vi "Untitled 9vi.vi"() -> ()   [LabVIEW 2009]
uses:
  <vilib>/Utility/file.llb/Read From Spreadsheet File (DBL).vi
  <vilib>/Analysis/NI_AALBase.lvlib
panel:
  in  "method":i32(ring)=1 items=["median", "noise center", "Minimum", "lower 20th"]
  out "white peaks":dbl
  out "white peaks normed":dbl
  out "red peaks normed":dbl
  in  "butterworth?":bool
  in  "w":dbl
  out "red peaks":dbl
  out "output cluster 3":cluster{"locations":dbl[], "locations":dbl[]}(graph)
  out "output cluster 2":cluster{"locations":dbl[], "amplitudes":dbl[]}[](graph)
  in  "threshold":dbl
  in  "number of rows (all:-1)":i32=300
  out "all rows":dbl[][](graph)
  in  "file path (dialog if empty)":path
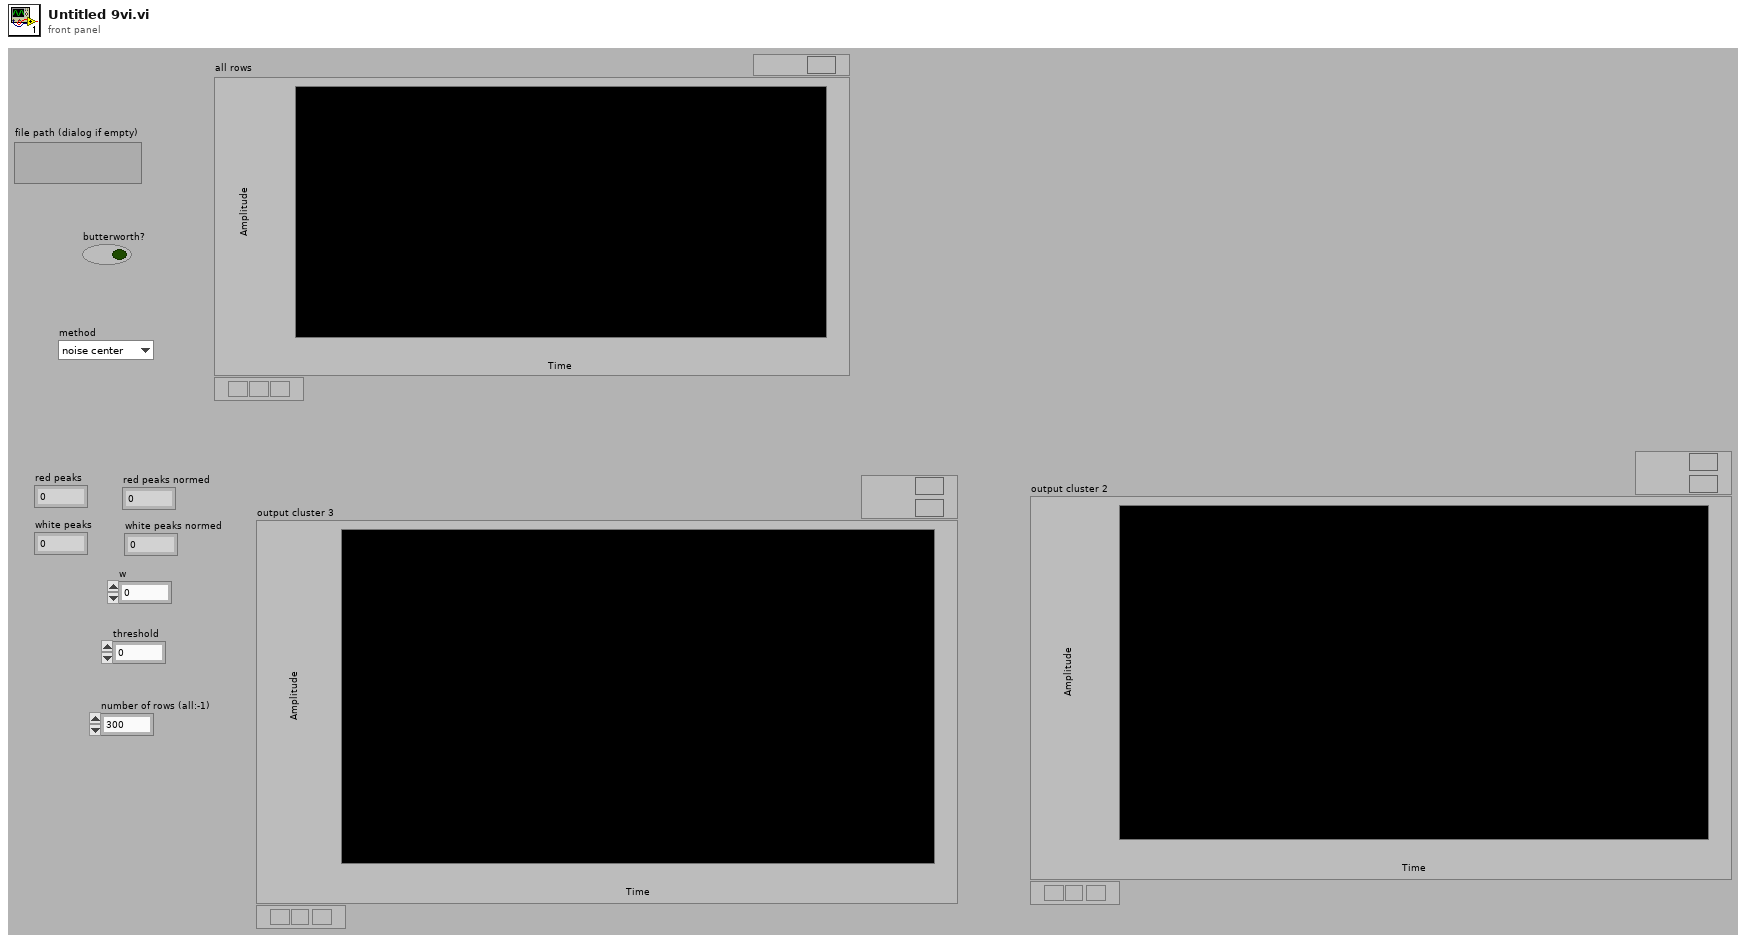
[diagram p1: front panel]
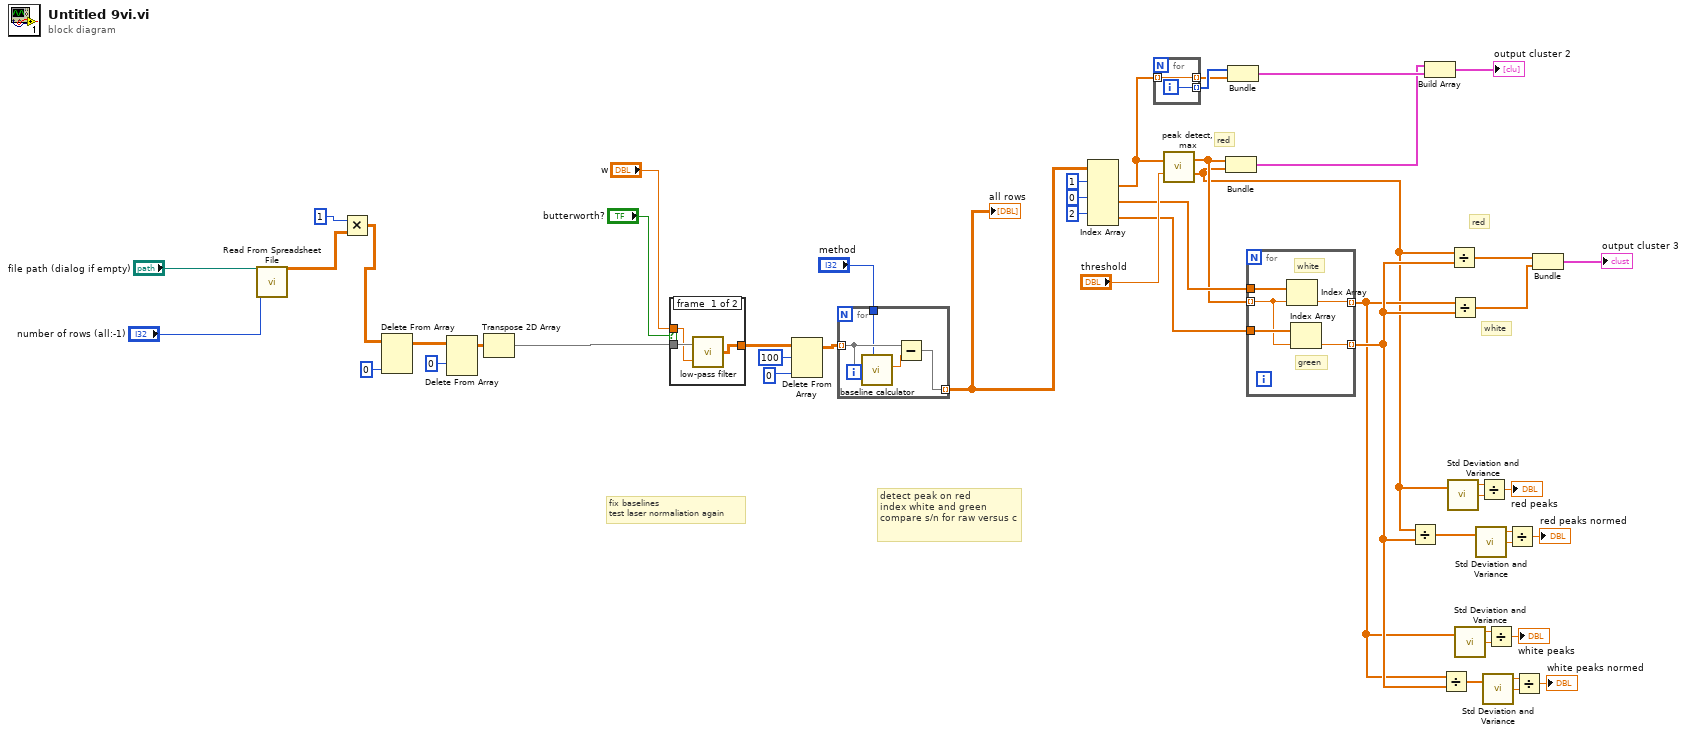
[diagram p0: block diagram]
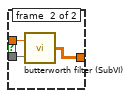
[diagram p2: hidden frame]
diagram:
  # "white"
  # "red"
  # "red"
  # "detect peak on red\nindex white and green\ncompare s/n for raw versus c"
  # "fix baselines\ntest laser normaliation again"
  n1 = call-poly <vilib>:"Read From Spreadsheet File.vi"("number of rows (all:-1)"="number of rows (all:-1)", "file path (dialog if empty)"="file path (dialog if empty)") -> ("all rows"=w44:dbl[][])  [unwired: 5 in, 4 out]
  n2 = Multiply(x=1 ("disabled index (col)"), y=w44) -> (x*y=w43:dbl[][])
  n3 = Delete From Array(array=w43, index (col)=0 ("disabled index (col)")) -> (array with subset deleted=w47:dbl[][])  [unwired: 2 in, 1 out]
  n4 = Delete From Array(array=w47, index (row)=0 ("disabled index (col)")) -> (array with subset deleted=w46:dbl[][])  [unwired: 2 in, 1 out]
  n5 = Transpose 2D Array(2D array=w46) -> (transposed array=w26:dbl[][])
  n6 = case shown="True" "butterworth?" {
    tunnel: "w" -> [w53 w57]
    tunnel: w26 -> [w54 w56]
    tunnel: [w52 w55] -> w12
    frame #0 {
      n7 = call "low-pass filter.vi"("smooth size"=w53, "Array 2"=w54) -> ("Array"=w52:dbl[][])
    }
    frame #1 {
      n8 = call "butterworth filter (SubVI).vi"("Array 2"=w56, "w"=w57) -> ("Array"=w55:dbl[][])
    }
  }
  n9 = Delete From Array(array=w12, length=100, index (col)=0 ("index (row)")) -> (array with subset deleted=w8:dbl[][])  [unwired: 1 in, 1 out]
  n10 = for {
    tunnel: w8 -> [w61] mode=indexing
    tunnel: [w59] -> w7 mode=indexing
    tunnel: "method" -> [w58]
    n11 = call "baseline calculator.vi"("method"=w58, "timetrace"=w61) -> ("baseline"=w60:dbl)  [unwired: 9 in]
    n12 = Subtract(x=w61, y=w60) -> (x-y=w59:dbl[])
  }
  "all rows" <- w7
  n13 = Index Array(array=w7, index (row) #1=1 ("disabled index (col)"), index (row) #2=0 ("disabled index (col)"), index (row) #3=2 ("index (row)")) -> (element #1=w33:dbl[], element #2=w32:dbl[], element #3=w20:dbl[])  [unwired: 3 in]
  n14 = for {
    tunnel: w33 -> [w63] mode=indexing
    tunnel: [w63] -> w34 mode=indexing
    tunnel: [w62] -> w35 mode=indexing
    i -> [w62]
  }
  n15 = call "peak detect, max.vi"("timetrace"=w33, "threshold"="threshold") -> ("locations"=w31:dbl[], "amplitudes"=w3:dbl[])  [unwired: 12 in]
  n16 = Bundle("locations"=w31, "amplitudes"=w3) -> (w37:cluster{"locations":dbl[], "amplitudes":dbl[]})  [unwired: 1 in]
  n17 = Bundle(w35, w34) -> (w38:cluster{i32[], dbl[]})  [unwired: 1 in]
  n18 = for {
    tunnel: w31 -> [w65] mode=indexing
    tunnel: w32 -> [w68]
    tunnel: [w67] -> w4 mode=indexing
    tunnel: w20 -> [w66]
    tunnel: [w64] -> w5 mode=indexing
    # "green"
    # "white"
    n19 = Index Array(array=w68, index=w65) -> (element=w67:dbl)
    n20 = Index Array(array=w66, index=w65) -> (element=w64:dbl)
  }
  n21 = Divide(x=w3, y=w5) -> (x/y=w9:dbl[])
  n22 = Build Array(w37, w38) -> (→"output cluster 2":cluster{"locations":dbl[], "amplitudes":dbl[]}[])
  n23 = Divide(x=w4, y=w5) -> (x/y=w19:dbl[])
  n24 = call <vilib>:"Std Deviation and Variance.vi"("X"=w3) -> ("mean"=w28:dbl, "standard deviation"=w29:dbl)  [unwired: 1 in, 1 out]
  n25 = Divide(x=w3, y=w5) -> (x/y=w1:dbl[])
  n26 = Divide(x=w4, y=w5) -> (x/y=w2:dbl[])
  n27 = call <vilib>:"Std Deviation and Variance.vi"("X"=w4) -> ("mean"=w15:dbl, "standard deviation"=w14:dbl)  [unwired: 1 in, 1 out]
  n28 = call <vilib>:"Std Deviation and Variance.vi"("X"=w9) -> ("mean"=w24:dbl, "standard deviation"=w23:dbl)  [unwired: 1 in, 1 out]
  n29 = Divide(x=w28, y=w29) -> (x/y=→"red peaks":dbl)
  n30 = call <vilib>:"Std Deviation and Variance.vi"("X"=w19) -> ("mean"=w16:dbl, "standard deviation"=w17:dbl)  [unwired: 1 in, 1 out]
  n31 = Divide(x=w15, y=w14) -> (x/y=→"white peaks":dbl)
  n32 = Divide(x=w24, y=w23) -> (x/y=→"red peaks normed":dbl)
  n33 = Divide(x=w16, y=w17) -> (x/y=→"white peaks normed":dbl)
  n34 = Bundle(w1, w2) -> (→"output cluster 3":cluster{dbl[], dbl[]})  [unwired: 1 in]
